vi "Load SCM Data.vi"(0 "# Records":i32=3, 1 "# Records to Skip":i32, 2 "Source File":path=path "C:/ScopeBinaryData.bin", 3 "# Channels":i32=7, 4 "Samples per Record":i32=51200) -> (5 "Array":dbl[][](array[numeric]))   [LabVIEW 2013]
panel:
  out "Size":i32[](array[numeric])
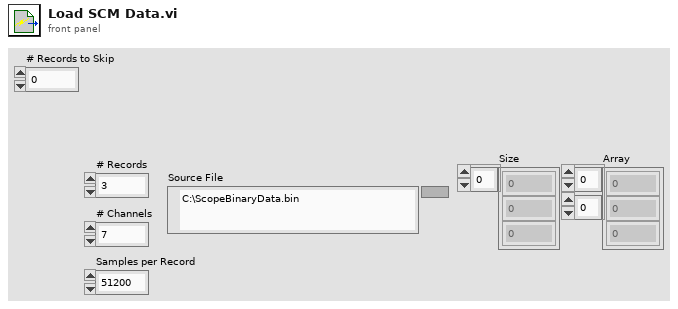
[diagram p1: front panel]
types:
  T1 = enum32{"CREATE_NEW (create)", "CREATE_ALWAYS (replace or create)", "OPEN_EXISTING (open)", "OPEN_ALWAYS (open or create)", "TRUNCATE_EXISTING (replace)"}
  T2 = enum16{"big-endian, network order", "native, host order", "little-endian"}
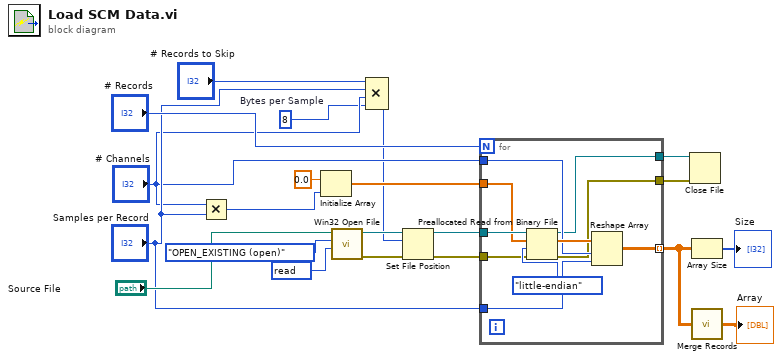
[diagram p0: block diagram]
diagram:
  w6 = 8  # Bytes per Sample
  w20 = u32 2147483648 items=["read"=2147483648, "write"=1073741824, "read & write"=3221225472, "execute"=536870912, "all"=268435456] ("desired access (read & write)")
  n1 = Multiply(x="# Channels", y="Samples per Record") -> (x*y=w15:i32)
  n2 = Initialize Array(0.0 ("element"), w15) -> (w16:dbl[])
  n3 = call "Win32 Open File.vi"("desired access (read & write)"=w20, "creation mode (open)"=T1."OPEN_EXISTING (open)", "file path"="Source File") -> ("error out"=w13:errorcluster, "LabVIEW file refnum out"=w12:refnum<file>)  [unwired: 6 in, 1 out]
  n4 = Compound Arithmetic op=MULTIPLY("# Records to Skip", "Samples per Record", "# Channels", w6) -> (w5:i32)
  n5 = Set File Position(offset (in bytes) (0)=w5, refnum=w12, error in=w13) -> (refnum out=w11:refnum<file>, error out=w10:errorcluster)  [unwired: 1 in]
  n6 = for {
    N: "# Records" -> [_]
    tunnel: w11 -> [w29]
    tunnel: w10 -> [w30]
    tunnel: w16 -> [w28]
    tunnel: "# Channels" -> [w26]
    tunnel: "Samples per Record" -> [w25]
    tunnel: [w24] -> w2 mode=indexing
    tunnel: [w23] -> w4
    tunnel: [w22] -> w3
    n7 = Preallocated Read from Binary File(4:w30, 5:T2."little-endian" ("byte order (0:big-endian, network order)"), 6:w28, 7:w29) -> (0:w22:errorcluster, 2:w27:dbl[], 3:w23:refnum<file>)  [unwired: 1 out]
    n8 = Reshape Array(w27, w26, w25) -> (w24:dbl[][])
  }
  n9 = Close File(refnum=w4, error in=w3) -> ()  [unwired: 2 out]
  n10 = Array Size(array=w2) -> (size(s)=→"Size":i32[])
  n11 = call "Merge Records.vi"("Records"=w2) -> ("Channel Data"=→"Array":dbl[][])  [unwired: 4 in]
